vi "DT2_discrete.vi"(0 "AI1":dbl, 1 "TD":dbl, 2 "Tcyc":dbl, 3 "D":dbl, 4 "f0":dbl, 5 "error in":errorcluster, 8 "Operation":T1(ring)) -> (16 "AO1":dbl, 19 "error out":errorcluster)   [LabVIEW 2022 SP3]
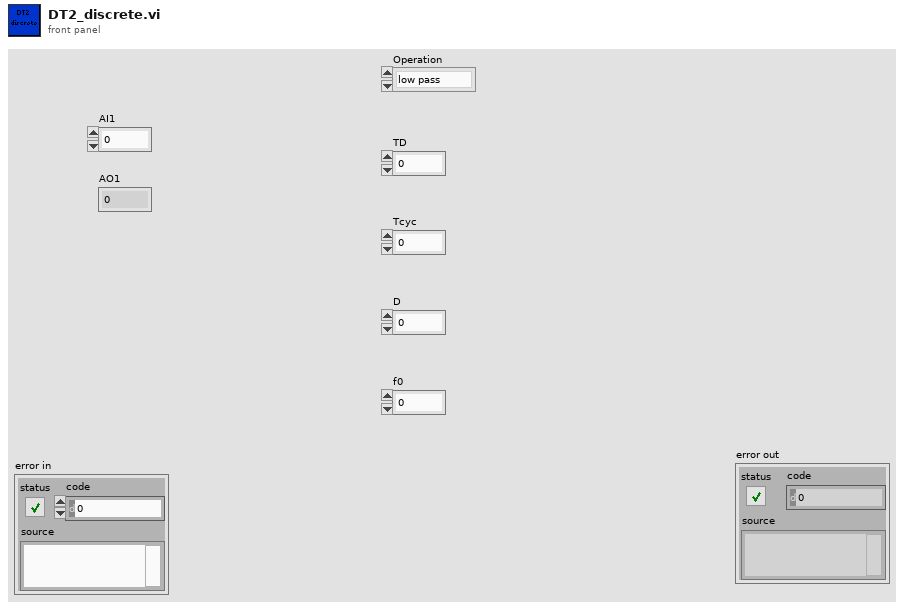
[diagram p1: front panel]
types:
  T1 = enum16{"low pass", "reset differentiation", "reset params"}
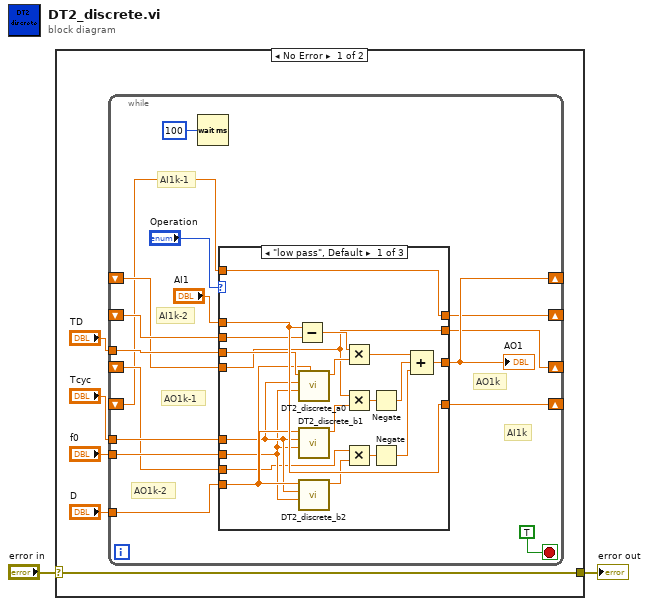
[diagram p0: block diagram]
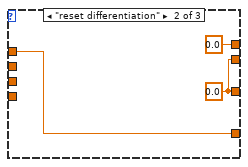
[diagram p2: hidden frame]
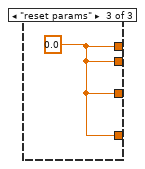
[diagram p3: hidden frame]
diagram:
  n1 = case shown="No Error" "error in" {
    selector: "error in" -> [w7 w47]
    tunnel: [w7 w47] -> w1
    frame No Error {
      n2 = while {
        shift-right: [w20] -> _
        shift-left: _ -> [w10]
        shift-right: [w9] -> _
        shift-left: _ -> [w19]
        tunnel: "D" -> [w18]
        tunnel: "TD" -> [w17]
        tunnel: "Tcyc" -> [w16]
        tunnel: "f0" -> [w15]
        shift-right: [w12] -> _
        shift-left: _ -> [w14]
        shift-right: [w8] -> _
        shift-left: _ -> [w13]
        stop <- TRUE stop-if-true
        # "AI1k-2"
        # "AO1k-2"
        # "AO1k-1"
        # "AI1k-1"
        # "AI1k"
        # "AO1k"
        n3 = Wait (ms)(milliseconds to wait=u32 100) -> ()  [unwired: 1 out]
        n4 = case shown="\"low pass\", Default" "Operation" {
          tunnel: [w42 w45 w46] -> w20
          tunnel: "AI1" -> [w42 w45 _]
          tunnel: w19 -> [w41 _ _]
          tunnel: w18 -> [w37 _ _]
          tunnel: w17 -> [w38 _ _]
          tunnel: w16 -> [w36 _ _]
          tunnel: w15 -> [w35 _ _]
          tunnel: w14 -> [w24 _ _]
          tunnel: w13 -> [w33 _ _]
          tunnel: [w26 w43 w46] -> w12
          tunnel: w10 -> [w25 _ _]
          tunnel: [w25 0.0 ("AI1") w46] -> w9
          tunnel: [w24 w43 w46] -> w8
          frame "low pass", Default {
            n5 = Subtract(x=w42, y=w41) -> (x-y=w40:dbl)
            n6 = call "DT2_discrete_a0.vi"("D"=w37, "f0"=w35, "Tcyc"=w36, "TD"=w38) -> ("a0"=w39:dbl)  [unwired: 6 in, 1 out]
            n7 = call "DT2_discrete_b1.vi"("f0"=w35, "Tcyc"=w36, "D"=w37) -> ("b1"=w34:dbl)  [unwired: 7 in, 1 out]
            n8 = call "DT2_discrete_b2.vi"("f0"=w35, "Tcyc"=w36, "D"=w37) -> ("b2"=w32:dbl)  [unwired: 7 in, 1 out]
            n9 = Multiply(x=w40, y=w39) -> (x*y=w31:dbl)
            n10 = Multiply(x=w24, y=w34) -> (x*y=w30:dbl)
            n11 = Multiply(x=w33, y=w32) -> (x*y=w28:dbl)
            n12 = Negate(x=w30) -> (-x=w29:dbl)
            n13 = Negate(x=w28) -> (-x=w27:dbl)
            n14 = Compound Arithmetic op=ADD(w31, w29, w27) -> (w26:dbl)
          }
          frame "reset differentiation" {
            w43 = 0.0
          }
          frame "reset params" {
            w46 = 0.0 ("AI1")
          }
        }
        "AO1" <- w12
      }
    }
    frame Error {
    }
  }
  "error out" <- w1
